vi "Select Action (SubVI).vi"(9 "State":i32, 11 "Q":dbl[][](array[numeric])) -> (3 "Action":i32)   [LabVIEW 2013]
doc: "Selects the action according to the Q and the current state. The action is selected according to the reward of the Q. The higher the reward is, the higher chance the correspoding action is selected.\n\nE.g. for a reward of 1 and 0, the possibility of selecting the 1st action is e/(e+1) and the 2nd is 1/(e+1)."
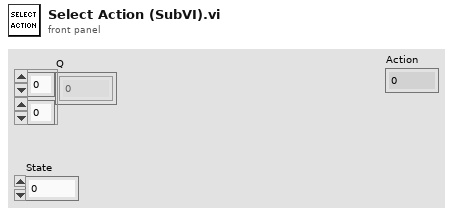
[diagram p1: front panel]
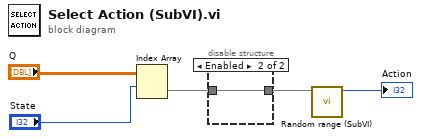
[diagram p0: block diagram]
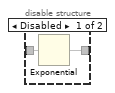
[diagram p2: hidden frame]
diagram:
  n1 = Index Array(array="Q", index (row)="State") -> (element=w3:dbl[])  [unwired: 1 in]
  n2 = disable-structure shown="Enabled" {
    disable-tunnel: w3 -> [w7 w8]
    disable-tunnel: [w6 w8] -> w2
    frame Disabled {
      n3 = Exponential(1:w7) -> (0:w6:dbl[])
    }
    frame Enabled {
    }
  }
  n4 = call "Random range (SubVI).vi"("Ranges"=w2) -> ("Index"=→"Action":i32)  [unwired: 9 in, 1 out]
